vi "IO.vi"() -> ()   [LabVIEW 2020]
uses:
  Global_Variable/Global.vi
  Libraries/S7/S7.lvlib
panel:
  in  "输入轴旋转手动速度":sgl caption="手动速度" format="%#.3f"
  in  "输入轴旋转-正转":bool
  in  "输入轴旋转-反转":bool
  in  "输入轴旋转绝对位置":sgl caption="绝对位置" format="%#.3f"
  in  "输入轴旋转相对位置":sgl caption="相对位置" format="%#.3f"
  in  "输入轴旋转-绝对定位":bool
  in  "输入轴旋转-相对定位":bool
  in  "输入轴移载手动速度":sgl caption="手动速度" format="%#.3f"
  in  "输入轴移载-正转":bool
  in  "输入轴移载-反转":bool
  in  "输入轴移载绝对位置":sgl caption="绝对位置" format="%#.3f"
  in  "输入轴移载相对位置":sgl caption="相对位置" format="%#.3f"
  in  "输入轴移载-绝对定位":bool
  in  "输入轴移载-相对定位":bool
  out "输出轴旋转当前位置":sgl caption="当前位置" format="%#.3f"
  in  "输出轴旋转-反转":bool
  in  "输出轴旋转-正转":bool
  in  "输出轴旋转手动速度":sgl caption="手动速度" format="%#.3f"
  in  "工装移载手动速度":sgl caption="手动速度" format="%#.3f"
  in  "工装移载-正转":bool
  in  "工装移载-反转":bool
  in  "工装移载绝对位置":sgl caption="绝对位置" format="%#.3f"
  in  "工装移载相对位置":sgl caption="相对位置" format="%#.3f"
  in  "工装移载-绝对定位":bool
  in  "工装移载-相对定位":bool
  out "输入轴旋转状态":bool
  out "输入轴移载状态":bool
  out "工装移载状态":bool
  out "输出轴旋转状态":bool
  in  "选项卡控件":enum32{"DI", "DO", "伺服"}(tab)
  out "I 1":T1
  out "I 3":T2
  out "I 2":T3
  out "I 0":T4
  out "I 4":T5
  out "I 5":T6
  in  "Q5":T7
  in  "Q4":T8
  in  "Q3":T9
  in  "Q2":T10
  in  "Q1":T11
  in  "Q0":T12
  out "吸收电流":sgl format="%#.3f"
  in  "Q6":T13
  out "输入扭矩":sgl format="%#.3f"
  out "输出扭矩(小)":sgl format="%#.3f"
  out "输出扭矩(大)":sgl format="%#.3f"
  out "输入轴旋转当前位置":sgl caption="当前位置" format="%#.3f"
  out "输入轴移载当前位置":sgl caption="当前位置" format="%#.3f"
  out "工装移载当前位置":sgl caption="当前位置" format="%#.3f"
  # "手动操作"
  # "输入轴旋转伺服"
  # "输出轴旋转伺服"
  # "输入轴移载伺服"
  # "工装移载伺服"
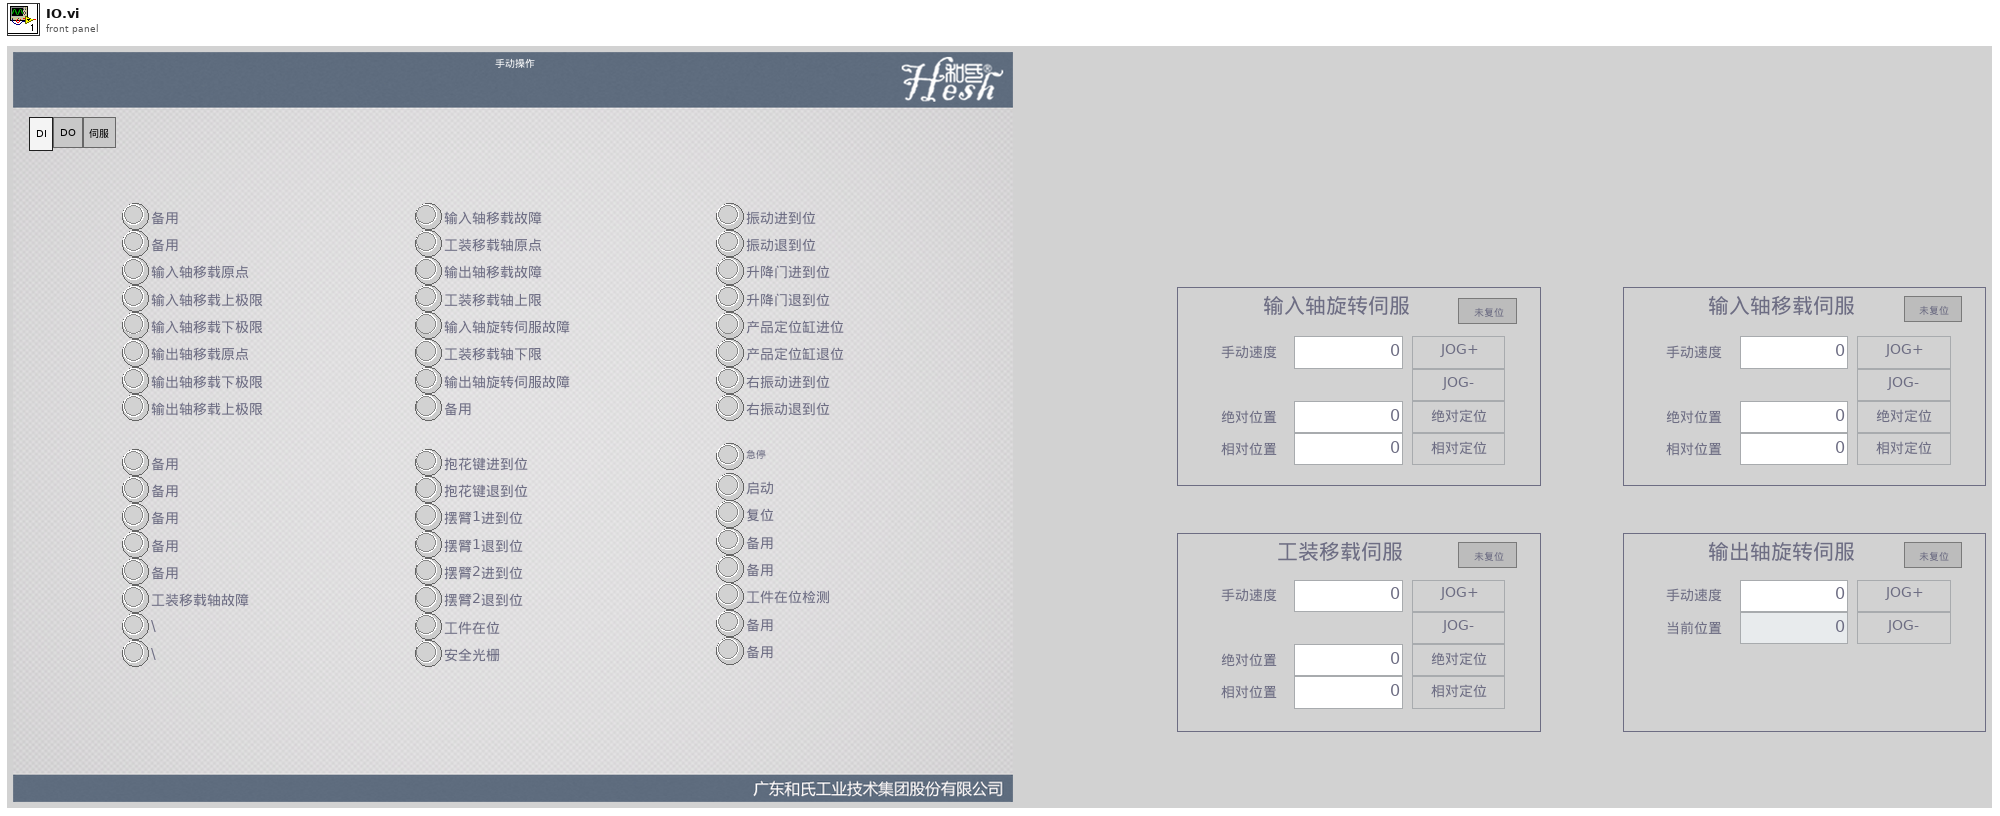
[diagram p1: front panel]
types:
  T1 = cluster{"备用":bool, "备用":bool, "备用":bool, "备用":bool, "备用":bool, "工装移载轴故障":bool, "\\":bool, "\\ ":bool}
  T2 = cluster{"抱花键进到位":bool, "抱花键退到位":bool, "摆臂1进到位":bool, "摆臂1退到位":bool, "摆臂2进到位":bool, "摆臂2退到位":bool, "工件在位":bool, "安全光栅":bool}
  T3 = cluster{"输入轴移载故障":bool, "工装移载轴原点":bool, "输出轴移载故障":bool, "工装移载轴上限":bool, "输入轴旋转伺服故障":bool, "工装移载轴下限":bool, "输出轴旋转伺服故障":bool, "备用":bool}
  T4 = cluster{"备用":bool, "备用":bool, "输入轴移载原点":bool, "输入轴移载上极限":bool, "输入轴移载下极限":bool, "输出轴移载原点":bool, "输出轴移载下极限":bool, "输出轴移载上极限":bool}
  T5 = cluster{"振动进到位":bool, "振动退到位":bool, "升降门进到位":bool, "升降门退到位":bool, "产品定位缸进位":bool, "产品定位缸退位":bool, "右振动进到位":bool, "右振动退到位":bool}
  T6 = cluster{"急停":bool, "启动":bool, "复位":bool, "备用":bool, "备用":bool, "工件在位检测":bool, "备用":bool, "备用":bool}
  T7 = cluster{"产品定位缸进":bool, "产品定位缸退":bool, "右振动进":bool, "右振动退":bool, "工装移载Reset":bool, "备用":bool, "工装移载JOG+":bool, "工装移载JOG-":bool}
  T8 = cluster{"抱花键":bool, "摆臂进":bool, "摆臂退":bool, "升降门进":bool, "升降门退":bool, "振动":bool, "电机方向":bool, "电机控制":bool}
  T9 = cluster{"三色灯黄":bool, "三色灯绿":bool, "三色灯红":bool, "蜂鸣器":bool, "备用":bool, "备用":bool, "备用":bool, "备用":bool}
  T10 = cluster{"输入轴移载Reset":bool, "输出轴移载Reset":bool, "输入轴旋转伺服启动":bool, "输入轴旋转伺服模式":bool, "输入轴旋转伺服Reset":bool, "输出轴旋转伺服启动":bool, "输出轴旋转伺服模式":bool, "输出轴旋转伺服Reset":bool}
  T11 = cluster{"工装移载Plus-":bool, "备用":bool, "/":bool, "/":bool, "/":bool, "/":bool, "/":bool, "/":bool}
  T12 = cluster{"输入轴移载Plus+":bool, "输入轴移载Plus-":bool, "输出轴移载Plus+":bool, "输出轴移载Plus-":bool, "模拟车速信号":bool, "控制器点火":bool, "模拟转速信号":bool, "工装移载Plus+":bool}
  T13 = cluster{"输入轴移载上升":bool, "输入轴移载下降":bool, "输出轴移载上升":bool, "输出轴移载下降":bool, "输入轴左旋":bool, "输入轴右旋":bool, "输出轴左旋":bool, "输出轴右旋":bool}
  T14 = cluster{bool, bool, bool, bool, bool, bool, bool, bool}
  T15 = typedef "S7.lvlib/Read_Data (Reply Payload)--cluster.ctl" = cluster{"读取成功":bool, "数据":u32[], "Read_Data_error":errorcluster}
  T16 = cluster{"Boolean array[0]":bool, "Boolean array[1]":bool, "Boolean array[2]":bool, "Boolean array[3]":bool, "Boolean array[4]":bool, "Boolean array[5]":bool, "Boolean array[6]":bool, "Boolean array[7]":bool}
  T17 = cluster{"输入旋转位移":sgl, "输入移载位移":sgl, "工装移载位移":sgl, "输入编码位移":sgl, "输入扭矩":sgl, "输出扭矩(小)":sgl, "输出扭矩(大)":sgl, "吸收电流":sgl, "Factorysensor":sgl, "输出轴旋转角度":sgl, "输出轴移栽位移":sgl, "Factorysensor2":sgl}
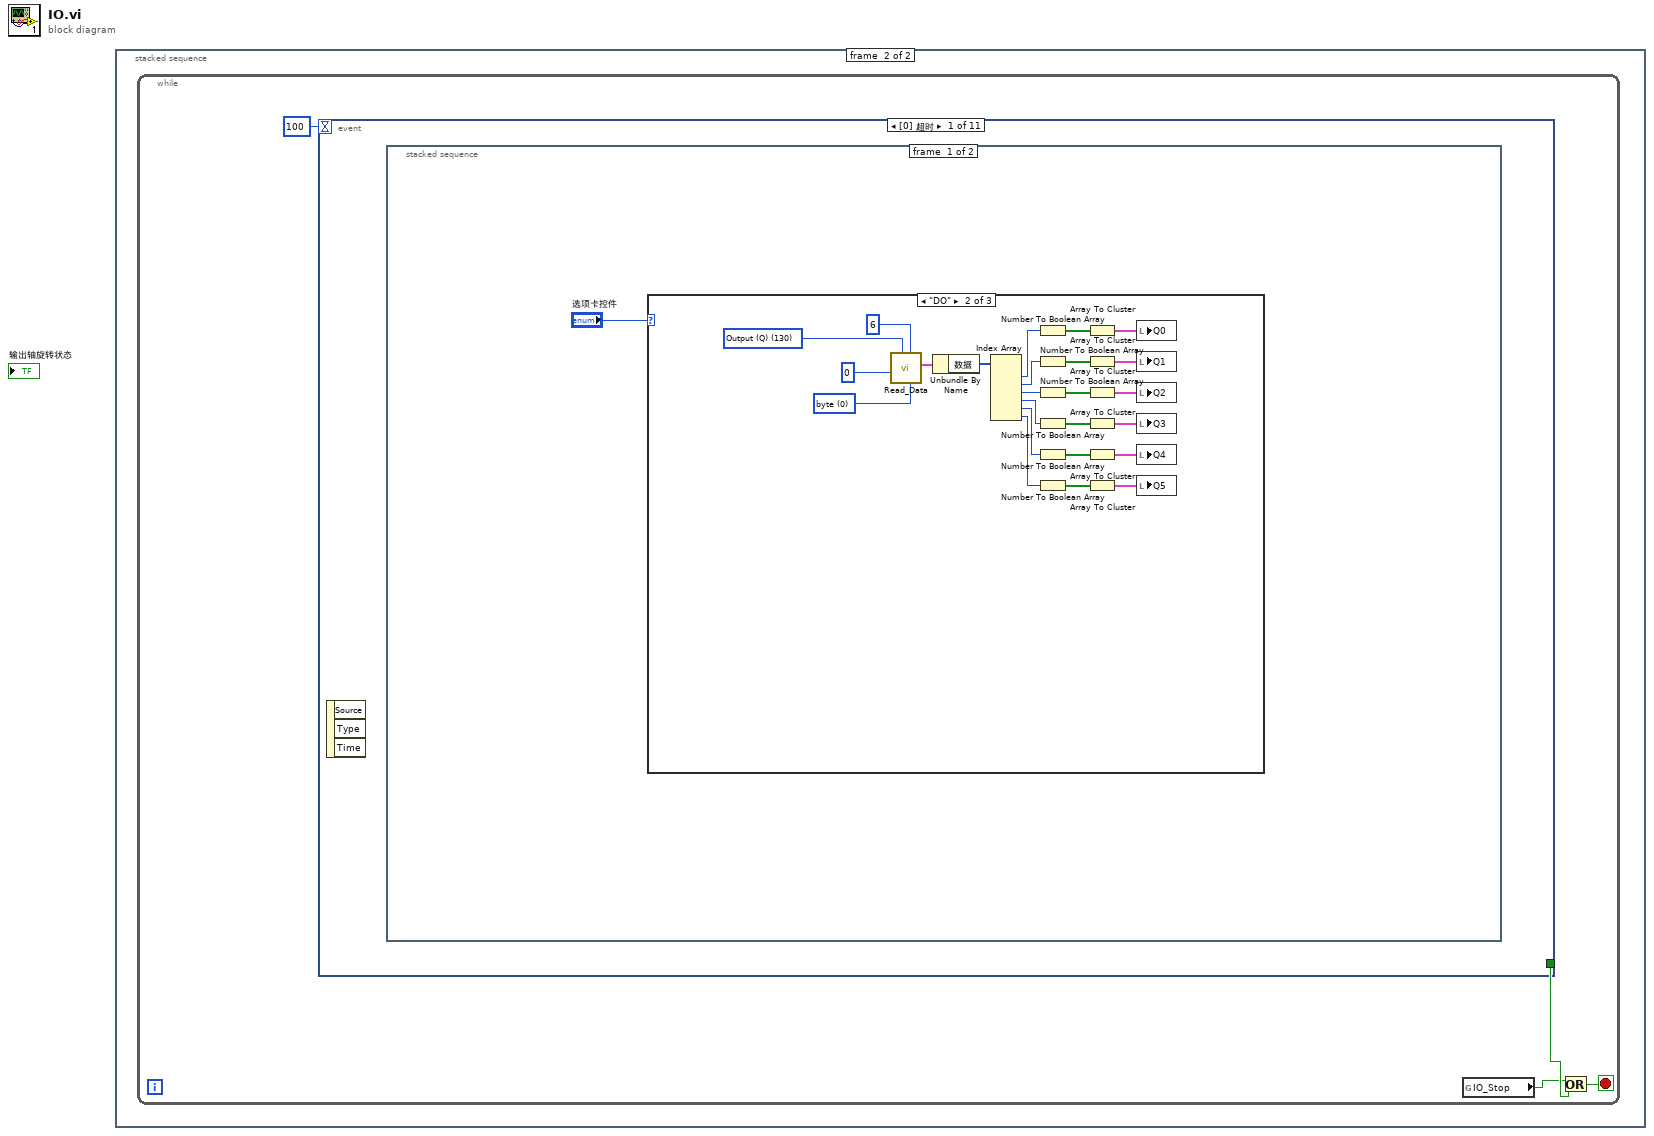
[diagram p0: block diagram]
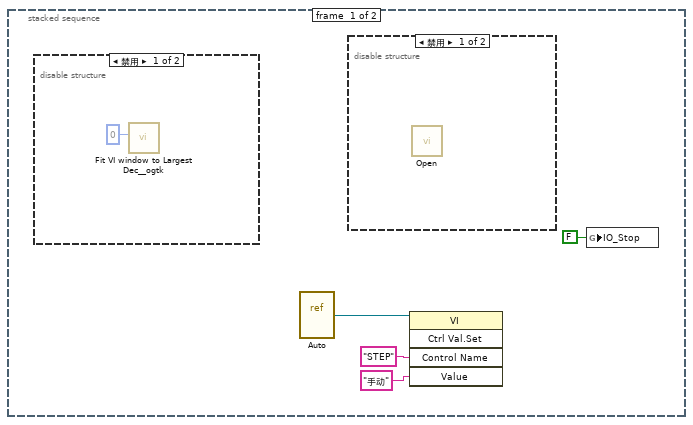
[diagram p2: hidden frame]
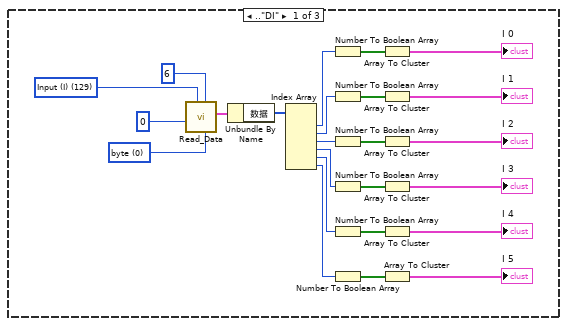
[diagram p5: hidden frame]
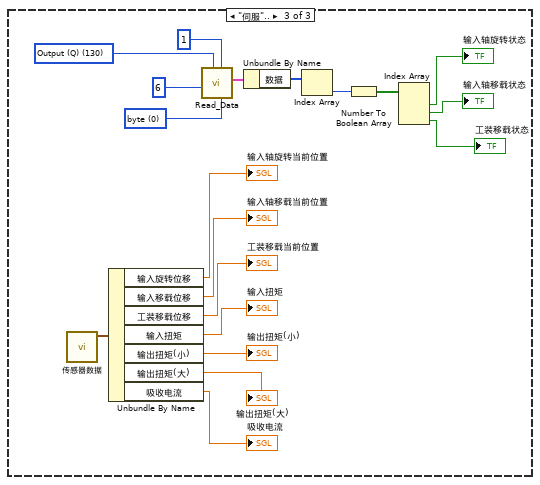
[diagram p6: hidden frame]
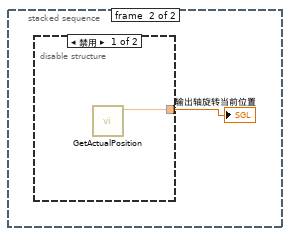
[diagram p7: hidden frame]
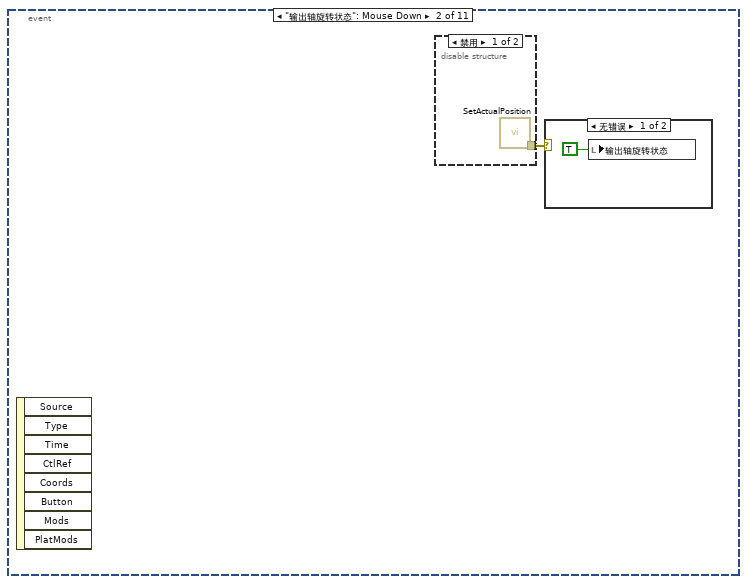
[diagram p9: hidden frame]
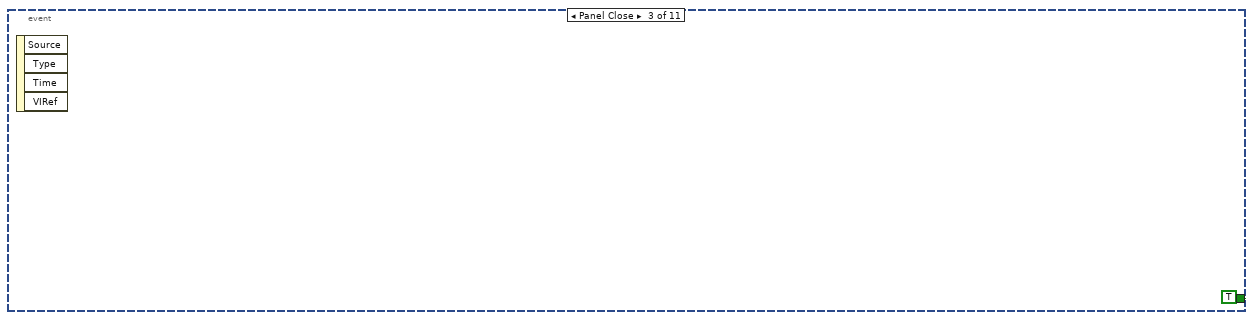
[diagram p12: hidden frame]
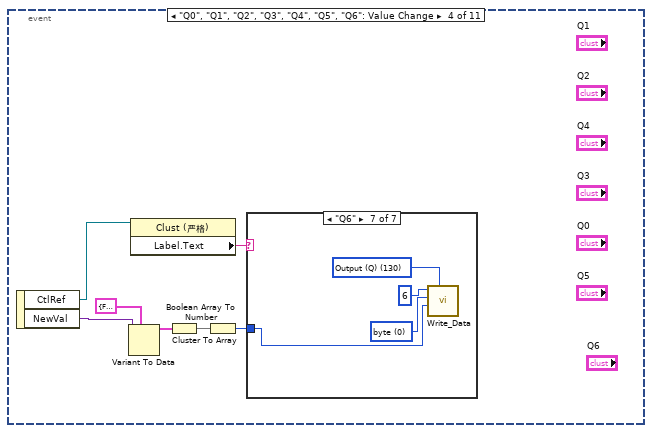
[diagram p13: hidden frame]
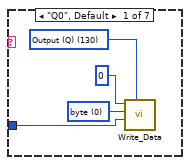
[diagram p14: hidden frame]
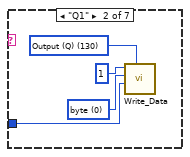
[diagram p15: hidden frame]
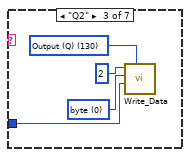
[diagram p16: hidden frame]
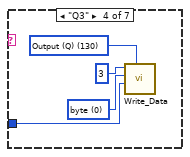
[diagram p17: hidden frame]
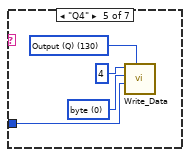
[diagram p18: hidden frame]
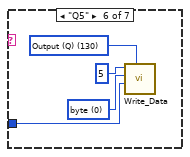
[diagram p19: hidden frame]
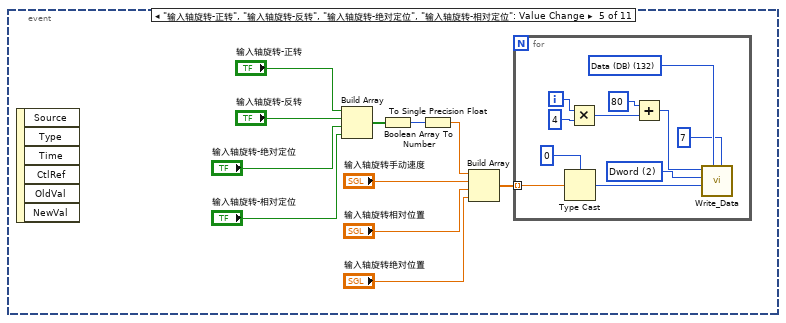
[diagram p20: hidden frame]
diagram:
  n1 = stacked-sequence {
    frame #0 {
      n2 = disable-structure shown="禁用" {
        frame Disabled {
          n3 = call <userlib>:"Fit VI window to Largest Dec__ogtk.vi"("border spacing (2 px)"=0) -> ()  [unwired: 5 in, 2 out]
        }
        frame Enabled {
        }
      }
      n4 = vi-ref "Auto.vi"() -> (w3:refnum<vi>)
      n5 = disable-structure shown="禁用" {
        frame Disabled {
          n6 = call "Open.vi"() -> ()  [unwired: 11 in, 1 out]
        }
        frame Enabled {
        }
      }
      n7 = invoke class="VI" method="Ctrl Val.Set"(reference=w3, "Control Name"="STEP" ("控件名"), "Value"="手动" ("控件名")) -> ()  [unwired: 2 in, 5 out]
      n8 = global write "Global.vi" "IO_Stop"(FALSE ("IO_Stop")) -> ()
    }
    frame #1 {
      n9 = while {
        stop <- w6 stop-if-true
        n10 = event shown="[0] 超时" {
          selector: _ -> [_ _ _ _ _ _ _ _ _ _ _]
          dyn-events: _ -> [_ _ _ _ _ _ _ _ _ _ _]
          timeout: 100 -> [_ _ _ _ _ _ _ _ _ _ _]
          tunnel: [_ _ TRUE _ _ _ _ _ _ _ _] -> w8
          event Timeout {
            n11 = event-data() -> ()  [unwired: 1 in, 3 out]
            n12 = stacked-sequence {
              frame #0 {
                n13 = case shown="\"DO\"" "选项卡控件" {
                  frame .."DI" {
                    w14 = u16 0 items=["byte", "word", "Dword"] ("数据类型")
                    w12 = u8 129 items=["I/O (P)"=128, "Input (I)"=129, "Output (Q)"=130, "Bit Memory (M)"=131, "Data (DB)"=132, "Instance Data (DI)"=133, "Local Data (L)"=134, "Predecessor Local Data (VL)"=135] ("寄存器类型")
                    n14 = call "Read_Data.vi"("数据类型"=w14, "读取长度"=u16 6, "寄存器类型"=w12, "起始地址"=u32 0) -> ("Reply Payload"=w16:T15)  [unwired: 5 in, 2 out]
                    n15 = Unbundle By Name(w16) -> ("数据"=w15:u32[])
                    n16 = Index Array(array=w15) -> (element #1=w28:u32, element #2=w30:u32, element #3=w29:u32, element #4=w25:u32, element #5=w24:u32, element #6=w23:u32)  [unwired: 6 in]
                    n17 = Number To Boolean Array(number=w28) -> (Boolean array=w27:bool[])
                    n18 = Number To Boolean Array(number=w30) -> (Boolean array=w26:bool[])
                    n19 = Number To Boolean Array(number=w29) -> (Boolean array=w22:bool[])
                    n20 = Number To Boolean Array(number=w25) -> (Boolean array=w20:bool[])
                    n21 = Number To Boolean Array(number=w24) -> (Boolean array=w18:bool[])
                    n22 = Number To Boolean Array(number=w23) -> (Boolean array=w17:bool[])
                    n23 = Array To Cluster(array=w27) -> (cluster=→"I 0":T16)
                    n24 = Array To Cluster(array=w26) -> (cluster=→"I 1":T16)
                    n25 = Array To Cluster(array=w22) -> (cluster=→"I 2":T16)
                    n26 = Array To Cluster(array=w20) -> (cluster=→"I 3":T16)
                    n27 = Array To Cluster(array=w18) -> (cluster=→"I 4":T16)
                    n28 = Array To Cluster(array=w17) -> (cluster=→"I 5":T16)
                  }
                  frame "DO" {
                    w38 = u16 0 items=["byte", "word", "Dword"] ("数据类型")
                    w36 = u8 130 items=["I/O (P)"=128, "Input (I)"=129, "Output (Q)"=130, "Bit Memory (M)"=131, "Data (DB)"=132, "Instance Data (DI)"=133, "Local Data (L)"=134, "Predecessor Local Data (VL)"=135] ("寄存器类型")
                    n29 = call "Read_Data.vi"("数据类型"=w38, "读取长度"=u16 6, "寄存器类型"=w36, "起始地址"=u32 0) -> ("Reply Payload"=w57:T15)  [unwired: 5 in, 2 out]
                    n30 = Unbundle By Name(w57) -> ("数据"=w58:u32[])
                    n31 = Index Array(array=w58) -> (element #1=w48:u32, element #2=w50:u32, element #3=w49:u32, element #4=w47:u32, element #5=w46:u32, element #6=w45:u32)  [unwired: 6 in]
                    n32 = Number To Boolean Array(number=w48) -> (Boolean array=w51:bool[])
                    n33 = Number To Boolean Array(number=w50) -> (Boolean array=w52:bool[])
                    n34 = Number To Boolean Array(number=w49) -> (Boolean array=w53:bool[])
                    n35 = Number To Boolean Array(number=w47) -> (Boolean array=w54:bool[])
                    n36 = Number To Boolean Array(number=w46) -> (Boolean array=w55:bool[])
                    n37 = Number To Boolean Array(number=w45) -> (Boolean array=w56:bool[])
                    n38 = Array To Cluster(array=w51) -> (cluster=w43:T16)
                    n39 = Array To Cluster(array=w52) -> (cluster=w44:T16)
                    n40 = Array To Cluster(array=w53) -> (cluster=w41:T16)
                    n41 = Array To Cluster(array=w54) -> (cluster=w42:T16)
                    n42 = Array To Cluster(array=w55) -> (cluster=w40:T16)
                    n43 = Array To Cluster(array=w56) -> (cluster=w39:T16)
                    n44 = local write "Q0"(w43) -> ()
                    n45 = local write "Q1"(w44) -> ()
                    n46 = local write "Q2"(w41) -> ()
                    n47 = local write "Q3"(w42) -> ()
                    n48 = local write "Q4"(w40) -> ()
                    n49 = local write "Q5"(w39) -> ()
                  }
                  frame "伺服".. {
                    w70 = u16 0 items=["byte", "word", "Dword"] ("数据类型")
                    w68 = u8 130 items=["I/O (P)"=128, "Input (I)"=129, "Output (Q)"=130, "Bit Memory (M)"=131, "Data (DB)"=132, "Instance Data (DI)"=133, "Local Data (L)"=134, "Predecessor Local Data (VL)"=135] ("寄存器类型")
                    n50 = call "传感器数据.vi"() -> ("传感器读数"=w62:T17)  [unwired: 10 in, 1 out]
                    n51 = Unbundle By Name(w62) -> ("输入旋转位移"=→"输入轴旋转当前位置":sgl, "输入移载位移"=→"输入轴移载当前位置":sgl, "工装移载位移"=→"工装移载当前位置":sgl, "输入扭矩"=→"输入扭矩":sgl, "输出扭矩(小)"=→"输出扭矩(小)":sgl, "输出扭矩(大)"=→"输出扭矩(大)":sgl, "吸收电流"=→"吸收电流":sgl)
                    n52 = call "Read_Data.vi"("数据类型"=w70, "读取长度"=u16 1, "寄存器类型"=w68, "起始地址"=u32 6) -> ("Reply Payload"=w71:T15)  [unwired: 5 in, 2 out]
                    n53 = Unbundle By Name(w71) -> ("数据"=w72:u32[])
                    n54 = Index Array(array=w72) -> (element=w77:u32)  [unwired: 1 in]
                    n55 = Number To Boolean Array(number=w77) -> (Boolean array=w74:bool[])
                    n56 = Index Array(array=w74) -> (element #1=→"输入轴旋转状态":bool, element #2=→"输入轴移载状态":bool, element #3=→"工装移载状态":bool)  [unwired: 3 in]
                  }
                }
              }
              frame #1 {
                n57 = disable-structure shown="禁用" {
                  disable-tunnel: [w79 _] -> w78
                  frame Disabled {
                    n58 = call "GetActualPosition.vi"() -> ("Axis_ActualPosition(°)"=w79:dbl)  [unwired: 11 in]
                  }
                  frame Enabled {
                  }
                }
                "输出轴旋转当前位置" <- w78
              }
            }
          }
          event "输出轴旋转状态": Mouse Down {
            n59 = event-data() -> ()  [unwired: 1 in, 8 out]
            n60 = disable-structure shown="禁用" {
              disable-tunnel: [w81 _] -> w80
              frame Disabled {
                n61 = call "SetActualPosition.vi"() -> ("error out"=w81:errorcluster)  [unwired: 11 in]
              }
              frame Enabled {
              }
            }
            n62 = case shown="无错误" w80 {
              frame No Error {
                n63 = local write "输出轴旋转状态"(TRUE ("输出轴旋转状态")) -> ()
              }
              frame Error {
              }
            }
          }
          event Panel Close {
            n64 = event-data() -> ()  [unwired: 1 in, 4 out]
          }
          event "Q0", "Q1", "Q2", "Q3", "Q4", "Q5", "Q6": Value Change {
            n65 = event-data() -> ("CtlRef"=w85:refnum<vi>, "NewVal"=w89:variant)  [unwired: 1 in]
            n66 = Variant To Data(type=T14 {FALSE, FALSE, FALSE, FALSE, FALSE, FALSE, FALSE, FALSE}, Variant=w89) -> (data=w88:T14)  [unwired: 1 in, 1 out]
            n67 = property class="Clust (严格)"(reference=w85) -> ("Label.Text"=w84:string)  [unwired: 1 in, 2 out]
            n68 = Cluster To Array(cluster=w88) -> (array=w87:bool[])
            n69 = Boolean Array To Number(Boolean array=w87) -> (number=w86:u32)
            n70 = case shown="\"Q6\"" w84 {
              tunnel: w86 -> [w94 w98 w102 w106 w110 w114 w115]
              frame "Q0", Default {
                w92 = u16 0 items=["byte", "word", "Dword"] ("数据类型")
                w93 = u8 130 items=["I/O (P)"=128, "Input (I)"=129, "Output (Q)"=130, "Bit Memory (M)"=131, "Data (DB)"=132, "Instance Data (DI)"=133, "Local Data (L)"=134, "Predecessor Local Data (VL)"=135] ("寄存器类型")
                n71 = call "Write_Data.vi"("寄存器类型"=w93, "写入数据"=w94, "数据类型"=w92, "写入地址"=u32 0) -> ()  [unwired: 5 in, 3 out]
              }
              frame "Q1" {
                w96 = u16 0 items=["byte", "word", "Dword"] ("数据类型")
                w97 = u8 130 items=["I/O (P)"=128, "Input (I)"=129, "Output (Q)"=130, "Bit Memory (M)"=131, "Data (DB)"=132, "Instance Data (DI)"=133, "Local Data (L)"=134, "Predecessor Local Data (VL)"=135] ("寄存器类型")
                n72 = call "Write_Data.vi"("寄存器类型"=w97, "写入数据"=w98, "数据类型"=w96, "写入地址"=u32 1) -> ()  [unwired: 5 in, 3 out]
              }
              frame "Q2" {
                w100 = u16 0 items=["byte", "word", "Dword"] ("数据类型")
                w101 = u8 130 items=["I/O (P)"=128, "Input (I)"=129, "Output (Q)"=130, "Bit Memory (M)"=131, "Data (DB)"=132, "Instance Data (DI)"=133, "Local Data (L)"=134, "Predecessor Local Data (VL)"=135] ("寄存器类型")
                n73 = call "Write_Data.vi"("寄存器类型"=w101, "写入数据"=w102, "数据类型"=w100, "写入地址"=u32 2) -> ()  [unwired: 5 in, 3 out]
              }
              frame "Q3" {
                w104 = u16 0 items=["byte", "word", "Dword"] ("数据类型")
                w105 = u8 130 items=["I/O (P)"=128, "Input (I)"=129, "Output (Q)"=130, "Bit Memory (M)"=131, "Data (DB)"=132, "Instance Data (DI)"=133, "Local Data (L)"=134, "Predecessor Local Data (VL)"=135] ("寄存器类型")
                n74 = call "Write_Data.vi"("寄存器类型"=w105, "写入数据"=w106, "数据类型"=w104, "写入地址"=u32 3) -> ()  [unwired: 5 in, 3 out]
              }
              frame "Q4" {
                w108 = u16 0 items=["byte", "word", "Dword"] ("数据类型")
                w109 = u8 130 items=["I/O (P)"=128, "Input (I)"=129, "Output (Q)"=130, "Bit Memory (M)"=131, "Data (DB)"=132, "Instance Data (DI)"=133, "Local Data (L)"=134, "Predecessor Local Data (VL)"=135] ("寄存器类型")
                n75 = call "Write_Data.vi"("寄存器类型"=w109, "写入数据"=w110, "数据类型"=w108, "写入地址"=u32 4) -> ()  [unwired: 5 in, 3 out]
              }
              frame "Q5" {
                w112 = u16 0 items=["byte", "word", "Dword"] ("数据类型")
                w113 = u8 130 items=["I/O (P)"=128, "Input (I)"=129, "Output (Q)"=130, "Bit Memory (M)"=131, "Data (DB)"=132, "Instance Data (DI)"=133, "Local Data (L)"=134, "Predecessor Local Data (VL)"=135] ("寄存器类型")
                n76 = call "Write_Data.vi"("寄存器类型"=w113, "写入数据"=w114, "数据类型"=w112, "写入地址"=u32 5) -> ()  [unwired: 5 in, 3 out]
              }
              frame "Q6" {
                w117 = u16 0 items=["byte", "word", "Dword"] ("数据类型")
                w118 = u8 130 items=["I/O (P)"=128, "Input (I)"=129, "Output (Q)"=130, "Bit Memory (M)"=131, "Data (DB)"=132, "Instance Data (DI)"=133, "Local Data (L)"=134, "Predecessor Local Data (VL)"=135] ("寄存器类型")
                n77 = call "Write_Data.vi"("寄存器类型"=w118, "写入数据"=w115, "数据类型"=w117, "写入地址"=u32 6) -> ()  [unwired: 5 in, 3 out]
              }
            }
          }
          event "输入轴旋转-正转", "输入轴旋转-反转", "输入轴旋转-绝对定位", "输入轴旋转-相对定位": Value Change {
            n78 = event-data() -> ()  [unwired: 1 in, 6 out]
            n79 = Build Array("输入轴旋转-正转", "输入轴旋转-反转", "输入轴旋转-绝对定位", "输入轴旋转-相对定位") -> (w128:bool[])
            n80 = Boolean Array To Number(Boolean array=w128) -> (number=w127:u32)
            n81 = To Single Precision Float(number=w127) -> (single precision float=w129:sgl)
            n82 = Build Array(w129, "输入轴旋转手动速度", "输入轴旋转相对位置", "输入轴旋转绝对位置") -> (w126:sgl[])
            n83 = for {
              tunnel: w126 -> [w135] mode=indexing
              i -> [w132]
              w137 = u16 2 items=["byte", "word", "Dword"] ("数据类型")
              w140 = u8 132 items=["I/O (P)"=128, "Input (I)"=129, "Output (Q)"=130, "Bit Memory (M)"=131, "Data (DB)"=132, "Instance Data (DI)"=133, "Local Data (L)"=134, "Predecessor Local Data (VL)"=135] ("寄存器类型")
              n84 = Type Cast(type=u32 0, x=w135) -> (*(type *) &x=w134:u32)
              n85 = Multiply(x=w132, y=u32 4) -> (x*y=w131:u32)
              n86 = Add(x=u32 80 ("写入地址"), y=w131) -> (x+y=w130:u32)
              n87 = call "Write_Data.vi"("DB #"=u16 7, "寄存器类型"=w140, "写入数据"=w134, "数据类型"=w137, "写入地址"=w130) -> ()  [unwired: 4 in, 3 out]
            }
          }
          event "输入轴移载-正转", "输入轴移载-反转", "输入轴移载-绝对定位", "输入轴移载-相对定位": Value Change {
            n88 = event-data() -> ()  [unwired: 1 in, 6 out]
            n89 = Build Array("输入轴移载-正转", "输入轴移载-反转", "输入轴移载-绝对定位", "输入轴移载-相对定位") -> (w150:bool[])
            n90 = Boolean Array To Number(Boolean array=w150) -> (number=w149:u32)
            n91 = To Single Precision Float(number=w149) -> (single precision float=w151:sgl)
            n92 = Build Array(w151, "输入轴移载手动速度", "输入轴移载相对位置", "输入轴移载绝对位置") -> (w148:sgl[])
            n93 = for {
              tunnel: w148 -> [w160] mode=indexing
              i -> [w158]
              w153 = u16 2 items=["byte", "word", "Dword"] ("数据类型")
              w155 = u8 132 items=["I/O (P)"=128, "Input (I)"=129, "Output (Q)"=130, "Bit Memory (M)"=131, "Data (DB)"=132, "Instance Data (DI)"=133, "Local Data (L)"=134, "Predecessor Local Data (VL)"=135] ("寄存器类型")
              n94 = Type Cast(type=u32 0, x=w160) -> (*(type *) &x=w152:u32)
              n95 = Multiply(x=w158, y=u32 4) -> (x*y=w157:u32)
              n96 = Add(x=u32 64 ("写入地址"), y=w157) -> (x+y=w154:u32)
              n97 = call "Write_Data.vi"("DB #"=u16 7, "寄存器类型"=w155, "写入数据"=w152, "数据类型"=w153, "写入地址"=w154) -> ()  [unwired: 4 in, 3 out]
            }
          }
          event "输出轴旋转-正转", "输出轴旋转-反转": Value Change {
            n98 = event-data() -> ()  [unwired: 1 in, 1 out]
            n99 = Build Array("输出轴旋转-正转", "输出轴旋转-反转") -> (w164:bool[])
            n100 = Boolean Array To Number(Boolean array=w164) -> (number=w163:u32)
            n101 = case shown="2" w163 {
              tunnel: "输出轴旋转手动速度" -> [_ w174 w175]
              tunnel: [sgl 0.0 ("输出轴旋转手动速度") w173 w175] -> w167
              frame 0, Default {
              }
              frame 2 {
                n102 = Negate(x=w174) -> (-x=w173:sgl)
              }
              frame 1 {
              }
            }
            n103 = disable-structure shown="禁用" {
              disable-tunnel: 100.0 ("Max Torque") -> [w171 _]
              disable-tunnel: w167 -> [w170 _]
              frame Disabled {
                n104 = call-poly "模式选择.vi"("Max Torque"=w171, "Velocity"=w170) -> ()  [unwired: 9 in, 1 out]
              }
              frame Enabled {
              }
            }
          }
          event "输入轴旋转状态": Mouse Down {
            w178 = u16 2 items=["byte", "word", "Dword"] ("数据类型")
            w180 = u8 132 items=["I/O (P)"=128, "Input (I)"=129, "Output (Q)"=130, "Bit Memory (M)"=131, "Data (DB)"=132, "Instance Data (DI)"=133, "Local Data (L)"=134, "Predecessor Local Data (VL)"=135] ("寄存器类型")
            n105 = event-data() -> ()  [unwired: 1 in, 1 out]
            n106 = Type Cast(type=u32 0, x=sgl 16.0) -> (*(type *) &x=w182:u32)
            n107 = call "Write_Data.vi"("DB #"=u16 7, "寄存器类型"=w180, "写入数据"=w182, "数据类型"=w178, "写入地址"=u32 80) -> ()  [unwired: 4 in, 3 out]
          }
          event "输入轴移载状态": Mouse Down {
            w183 = u16 2 items=["byte", "word", "Dword"] ("数据类型")
            w186 = u8 132 items=["I/O (P)"=128, "Input (I)"=129, "Output (Q)"=130, "Bit Memory (M)"=131, "Data (DB)"=132, "Instance Data (DI)"=133, "Local Data (L)"=134, "Predecessor Local Data (VL)"=135] ("寄存器类型")
            n108 = event-data() -> ()  [unwired: 1 in, 1 out]
            n109 = Type Cast(type=u32 0, x=sgl 16.0) -> (*(type *) &x=w189:u32)
            n110 = call "Write_Data.vi"("DB #"=u16 7, "寄存器类型"=w186, "写入数据"=w189, "数据类型"=w183, "写入地址"=u32 64) -> ()  [unwired: 4 in, 3 out]
          }
          event "工装移载状态": Mouse Down {
            w190 = u16 2 items=["byte", "word", "Dword"] ("数据类型")
            w193 = u8 132 items=["I/O (P)"=128, "Input (I)"=129, "Output (Q)"=130, "Bit Memory (M)"=131, "Data (DB)"=132, "Instance Data (DI)"=133, "Local Data (L)"=134, "Predecessor Local Data (VL)"=135] ("寄存器类型")
            n111 = event-data() -> ()  [unwired: 1 in, 1 out]
            n112 = Type Cast(type=u32 0, x=sgl 16.0) -> (*(type *) &x=w196:u32)
            n113 = call "Write_Data.vi"("DB #"=u16 7, "寄存器类型"=w193, "写入数据"=w196, "数据类型"=w190, "写入地址"=u32 104) -> ()  [unwired: 4 in, 3 out]
          }
          event "工装移载-正转", "工装移载-反转", "工装移载-绝对定位", "工装移载-相对定位": Value Change {
            n114 = event-data() -> ()  [unwired: 1 in, 6 out]
            n115 = Build Array("工装移载-正转", "工装移载-反转", "工装移载-绝对定位", "工装移载-相对定位") -> (w203:bool[])
            n116 = Boolean Array To Number(Boolean array=w203) -> (number=w202:u32)
            n117 = To Single Precision Float(number=w202) -> (single precision float=w201:sgl)
            n118 = Build Array(w201, "工装移载手动速度", "工装移载相对位置", "工装移载绝对位置") -> (w199:sgl[])
            n119 = for {
              tunnel: w199 -> [w213] mode=indexing
              i -> [w210]
              w215 = u16 2 items=["byte", "word", "Dword"] ("数据类型")
              w218 = u8 132 items=["I/O (P)"=128, "Input (I)"=129, "Output (Q)"=130, "Bit Memory (M)"=131, "Data (DB)"=132, "Instance Data (DI)"=133, "Local Data (L)"=134, "Predecessor Local Data (VL)"=135] ("寄存器类型")
              n120 = Type Cast(type=u32 0, x=w213) -> (*(type *) &x=w212:u32)
              n121 = Multiply(x=w210, y=u32 4) -> (x*y=w209:u32)
              n122 = Add(x=u32 104 ("写入地址"), y=w209) -> (x+y=w208:u32)
              n123 = call "Write_Data.vi"("DB #"=u16 7, "寄存器类型"=w218, "写入数据"=w212, "数据类型"=w215, "写入地址"=w208) -> ()  [unwired: 4 in, 3 out]
            }
          }
        }
        n124 = global read "Global.vi" "IO_Stop"() -> (w7:bool)
        n125 = Or(x=w7, y=w8) -> (x .or. y?=w6:bool)
      }
    }
  }
